vi "FL_Last_N_Samples_1D_for_waveforms.vi"(1 "BufferLengthSamples":u32=640, 2 "Mouse speed input":dbl caption="Mouse speed" format="%05.1f", 3 "Input timestamp":timestamp) -> (0 "Output waveform":waveform(dbl))   [LabVIEW 2018]
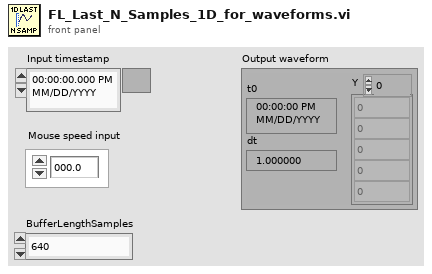
[diagram p1: front panel]
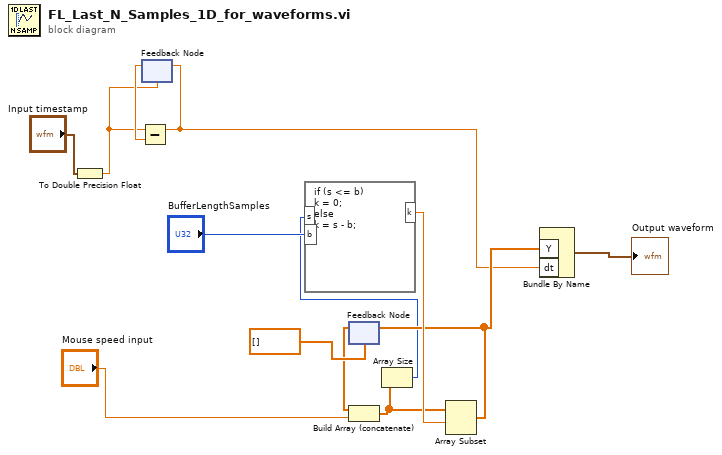
[diagram p0: block diagram]
diagram:
  n1 = To Double Precision Float(number="Input timestamp") -> (double precision float=w5:dbl)
  n2 = feedback #1(w5) -> (w7:dbl)
  n3 = Subtract(x=w5, y=w7) -> (x-y=w2:dbl)
  n4 = feedback-in #1(w2) -> ()
  n5 = feedback #2(dbl[] []) -> (w11:dbl[])
  n6 = Build Array (concatenate)(w11, "Mouse speed input") -> (w4:dbl[])
  n7 = Array Size(array=w4) -> (size(s)=w3:i32)
  n8 = formula code="if (s <= b)\nk = 0;\nelse\nk = s - b;"("s"=w3, "b"="BufferLengthSamples") -> ("k"=w9:dbl)
  n9 = Array Subset(array=w4, index=w9) -> (w8:dbl[])  [unwired: 1 in]
  n10 = feedback-in #2(w8) -> ()
  n11 = Bundle By Name("Y"=w8, "dt"=w2) -> (→"Output waveform":waveform(dbl))  [unwired: 1 in]
